vi "init.vi"(10 "ZC-Generation options":T1={"Sequence length"=64, "Sequence Root"=25, "# of subcarriers"=31, "Amplitude"=8.0, "Decimation Factor"=8, "Threshold"=20.0} {"Decimation Factor" min=1 max=8 step=1}) -> (0 "error out":errorcluster, 3 "Synchronizer out":refnum<class "Synchronizer.lvclass">)   [LabVIEW 2012, in "Synchronizer.lvclass"]
uses:
  Synchronizer.lvclass
  Synchronizer.lvclass/Synchronizer.ctl
  <vilib>/imath/engines/lvmath2/RunTimeEngine/ErrorHandling/NIMS_Finalize Error.vi
  <vilib>/imath/engines/lvmath2/RunTimeEngine/Managers/WorkSpace/UID Generator.vi
  <vilib>/imath/engines/lvmath2/RunTimeEngine/BuiltInFunctions/zeros/NIMS_V=zeros(I32,I32).vi
  <vilib>/imathl/engines/lvmath/Functions/Error Handling/Create Error.vi
  <vilib>/imath/engines/lvmath2/RunTimeEngine/RangeToken/NIMS_Range_R2 - Integer.vi
  <instcachedir>/0/NIMS_Range_R2 - Integer_CD92A44154CA48D58B2F3E711AB114DB.lvgen/NIMS_Range_R2 - Integer_CD92A44154CA48D58B2F3E711AB114DB_000.vi
  <vilib>/imath/engines/lvmath2/RunTimeEngine/Managers/SymbolTable/Clear UID.vi
  <vilib>/imath/engines/lvmath2/RunTimeEngine/NodeEndStatement/NIMS_NodeEndStatement_Output.vi
  <instcachedir>/0/NIMS_NodeEndStatement_Output_53EC0D466D134D7ABD903AC30B43404B.lvgen/NIMS_NodeEndStatement_Output_53EC0D466D134D7ABD903AC30B43404B_000.vi
  <vilib>/imath/engines/lvmath2/RunTimeEngine/CommandStatement/MC_CommandStatement_break.vi
  <vilib>/imath/engines/lvmath2/RunTimeEngine/RunTimeType/NIMS_RunTimeType_From StrictType (excl LVString).vi
  <instcachedir>/0/NIMS_RunTimeType_From StrictType (excl LVString)_AC52D965D0864706932D20A05968E122.lvgen/NIMS_RunTimeType_From StrictType (excl LVString)_AC52D965D0864706932D20A05968E122_000.vi
  <vilib>/imath/engines/lvmath2/RunTimeEngine/LocalVariableDefStatement/MC_LocalVariableDefStatement_Display.vi
  <vilib>/imath/engines/lvmath2/RunTimeEngine/ReplaceToken/NIMS_Replace - Check Linear.vi
  <instcachedir>/0/NIMS_Replace - Check Linear_44ABB4D6A819426DBDF25CCE6827BF1D.lvgen/NIMS_Replace - Check Linear_44ABB4D6A819426DBDF25CCE6827BF1D_002.vi
  <vilib>/imath/engines/lvmath2/RunTimeEngine/ReplaceToken/NIMS_Replace - Size Check _(_)=S.vi
  <instcachedir>/0/NIMS_Replace - Size Check _(_)=S_5AC8AA27B9694BB9828B57BCF666F597.lvgen/NIMS_Replace - Size Check _(_)=S_5AC8AA27B9694BB9828B57BCF666F597_001.vi
  <vilib>/imath/engines/lvmath2/RunTimeEngine/ReplaceToken/NIMS_Replace - V(S)=S.vi
  <instcachedir>/0/NIMS_Replace - V(S)=S_927EF1B21AA84780A9A306EC96B904EC.lvgen/NIMS_Replace - V(S)=S_927EF1B21AA84780A9A306EC96B904EC_001.vi
  <vilib>/imath/engines/lvmath2/RunTimeEngine/BuiltInFunctions/reverse_vector/NIMS_reverse_vector(GV).vi
  <instcachedir>/0/NIMS_reverse_vector(GV)_EC0BA47EA39D43F9B3C4AC54DC888C76.lvgen/NIMS_reverse_vector(GV)_EC0BA47EA39D43F9B3C4AC54DC888C76_004.vi
  <vilib>/imath/engines/lvmath2/RunTimeEngine/BuiltInFunctions/ifft/NIMS_ifft(CV).vi
  <vilib>/imath/engines/lvmath2/RunTimeEngine/ErrorHandling/NIMS_Error From Error Code.vi
  <vilib>/imath/engines/lvmath2/RunTimeEngine/BuiltInFunctions/conjugate/NIMS_conjugate(Complex).vi
  <instcachedir>/0/NIMS_conjugate(Complex)_151E186CA54B4853A0120BB0A667D86E.lvgen/NIMS_conjugate(Complex)_151E186CA54B4853A0120BB0A667D86E_001.vi
  <vilib>/imath/engines/lvmath2/RunTimeEngine/Managers/SymbolTable/NIMS_WorkSpace.lvlib
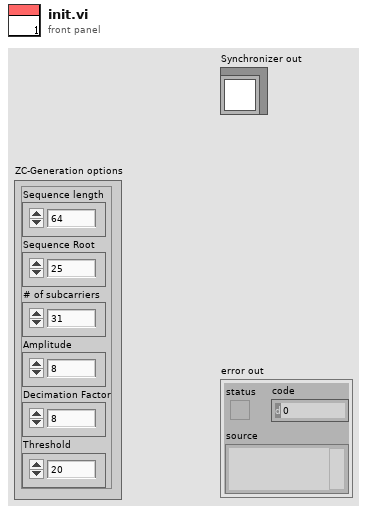
[diagram p1: front panel]
types:
  T1 = cluster{"Sequence length":i32, "Sequence Root":i32, "# of subcarriers":i32, "Amplitude":dbl, "Decimation Factor":u8, "Threshold":dbl}
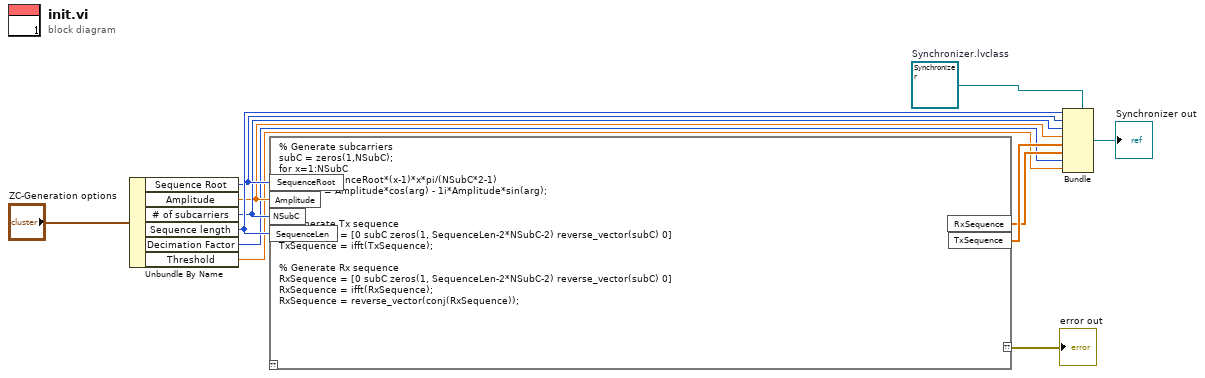
[diagram p0: block diagram]
diagram:
  w11 = refnum<class "Synchronizer.lvclass"> refnum  # Synchronizer.lvclass
  n1 = Unbundle By Name("ZC-Generation options") -> ("Sequence Root"=w5:i32, "Amplitude"=w3:dbl, "# of subcarriers"=w4:i32, "Sequence length"=w6:i32, "Decimation Factor"=w2:u8, "Threshold"=w1:dbl)
  n2 = mathscript code="% Generate subcarriers\nsubC = zeros(1,NSubC);\nfor x=1:NSubC\n  arg = SequenceRoot*(x-1)*x*pi/(NSubC*2-1)\n  subC(x) = Amplitude*cos(arg) - 1i*Amplitude*sin(arg);\nend\n\n% Generate Tx sequence\nTxSequence = [0 subC zeros(1, SequenceLen-2*NSubC-2) reverse_vector(subC) 0]\nTxSequence = ifft(TxSequence);\n\n% Generate Rx sequence\nRxSequence = [0 subC zeros(1, SequenceLen-2*NSubC-2) reverse_vector(subC) 0]\nRxSequence = ifft(RxSequence);\nRxSequence = reverse_vector(conj(RxSequence));"("SequenceRoot"=w5, "NSubC"=w4, "SequenceLen"=w6, "Amplitude"=w3) -> ("??"=→"error out":errorcluster, "RxSequence"=w8:cdb[], "TxSequence"=w9:cdb[])  [unwired: 1 in]
  n3 = Bundle(cluster=w11, w6, w5, w4, w3, w9, w8, w2, w1) -> (→"Synchronizer out":refnum<class "Synchronizer.lvclass">)
